vi "Cieslikiewicz_prac10.vi"() -> ()   [LabVIEW 2023]
uses:
  <vilib>/Platform/TimedLoop/XDataNode/timing_clust.ctl
  <vilib>/Platform/TimedLoop/XDataNode/nitl_modes.ctl
  <vilib>/Platform/TimedLoop/XDataNode/wakeup.ctl
  <vilib>/Platform/TimedLoop/scheduler/LVUserAPI/_suppVIs/Create_1kHz_TSource.vi
  <vilib>/platform/TimedLoop/XDataNode/XDataNode.xnode
  <vilib>/Platform/TimedLoop/XDataNode/XDNodeRunTimeDep.lvlib
panel:
  in  "Synchronizacja":bool
  out "L2 Stop":dbl
  out "Error 2":errorcluster
  out "Koniec 2":bool
  out "L2 End":dbl
  out "Numer petli 2":dbl
  out "L1 Stop":dbl
  out "czas_pocz":dbl
  out "Koniec 1":bool
  out "Error 1":errorcluster
  out "Numer petli 1":dbl
  out "L1 End":dbl
  in  "Okres (s)":dbl=0.5 min=0.5 max=20.0 step=0.5
  out "S0 End":dbl
  out "S0 Start":dbl
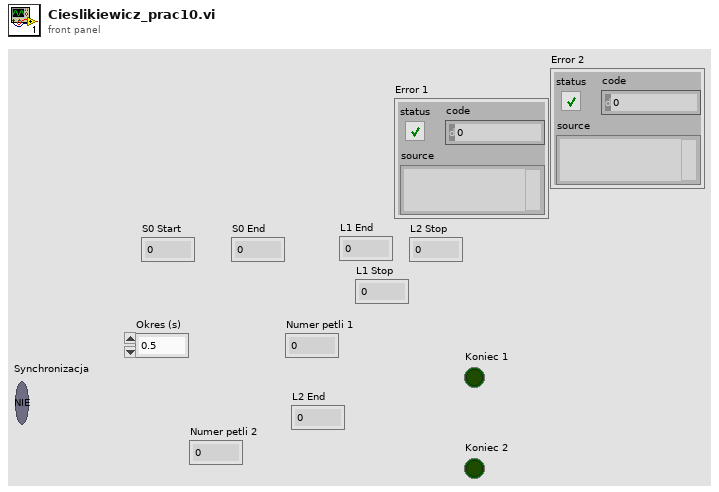
[diagram p1: front panel]
types:
  T1 = typedef "XDNodeRunTimeDep.lvlib/timing_clust.ctl" = cluster{"Expected End [f-1]":u64, "Actual End [f-1]":u64, "Finished Late? [f-1]":bool, "Expected End [i-1]":u64, "Actual End [i-1]":u64, "Finished Late? [i-1]":bool, "Expected Start [i]":u64, "Actual Start [i]":u64, "Expected Start [f]":u64, "Actual Start [f]":u64, "Source Name":string, "Structure Name":string, "Period":i64, "Deadline":i64, "Offset":i64, "Start":i64, "Priority":i32, "Timeout":i32, "Mode":T2, "Wakeup Reason":T3, "Error":errorcluster, "Source Type":string, "Secondary Source Type":string, "Global End Time":u64, "Global Start Time":u64, "Frame Duration":u64, "Iteration Duration":u64, "Assigned CPU":i32, "I/O Scan Engine Mode":u32}
  T2 = typedef "XDNodeRunTimeDep.lvlib/nitl_modes.ctl" = enum32{"No Change", "Process missed periods, maintain original phase", "Discard missed periods, maintain original phase", "Process missed periods, ignore original phase", "Discard missed periods, ignore original phase"}
  T3 = typedef "XDNodeRunTimeDep.lvlib/wakeup.ctl" = enum32{"Normal", "Aborted", "Asynchronous wakeup", "Timing source error", "Timed loop error", "Timeout"}
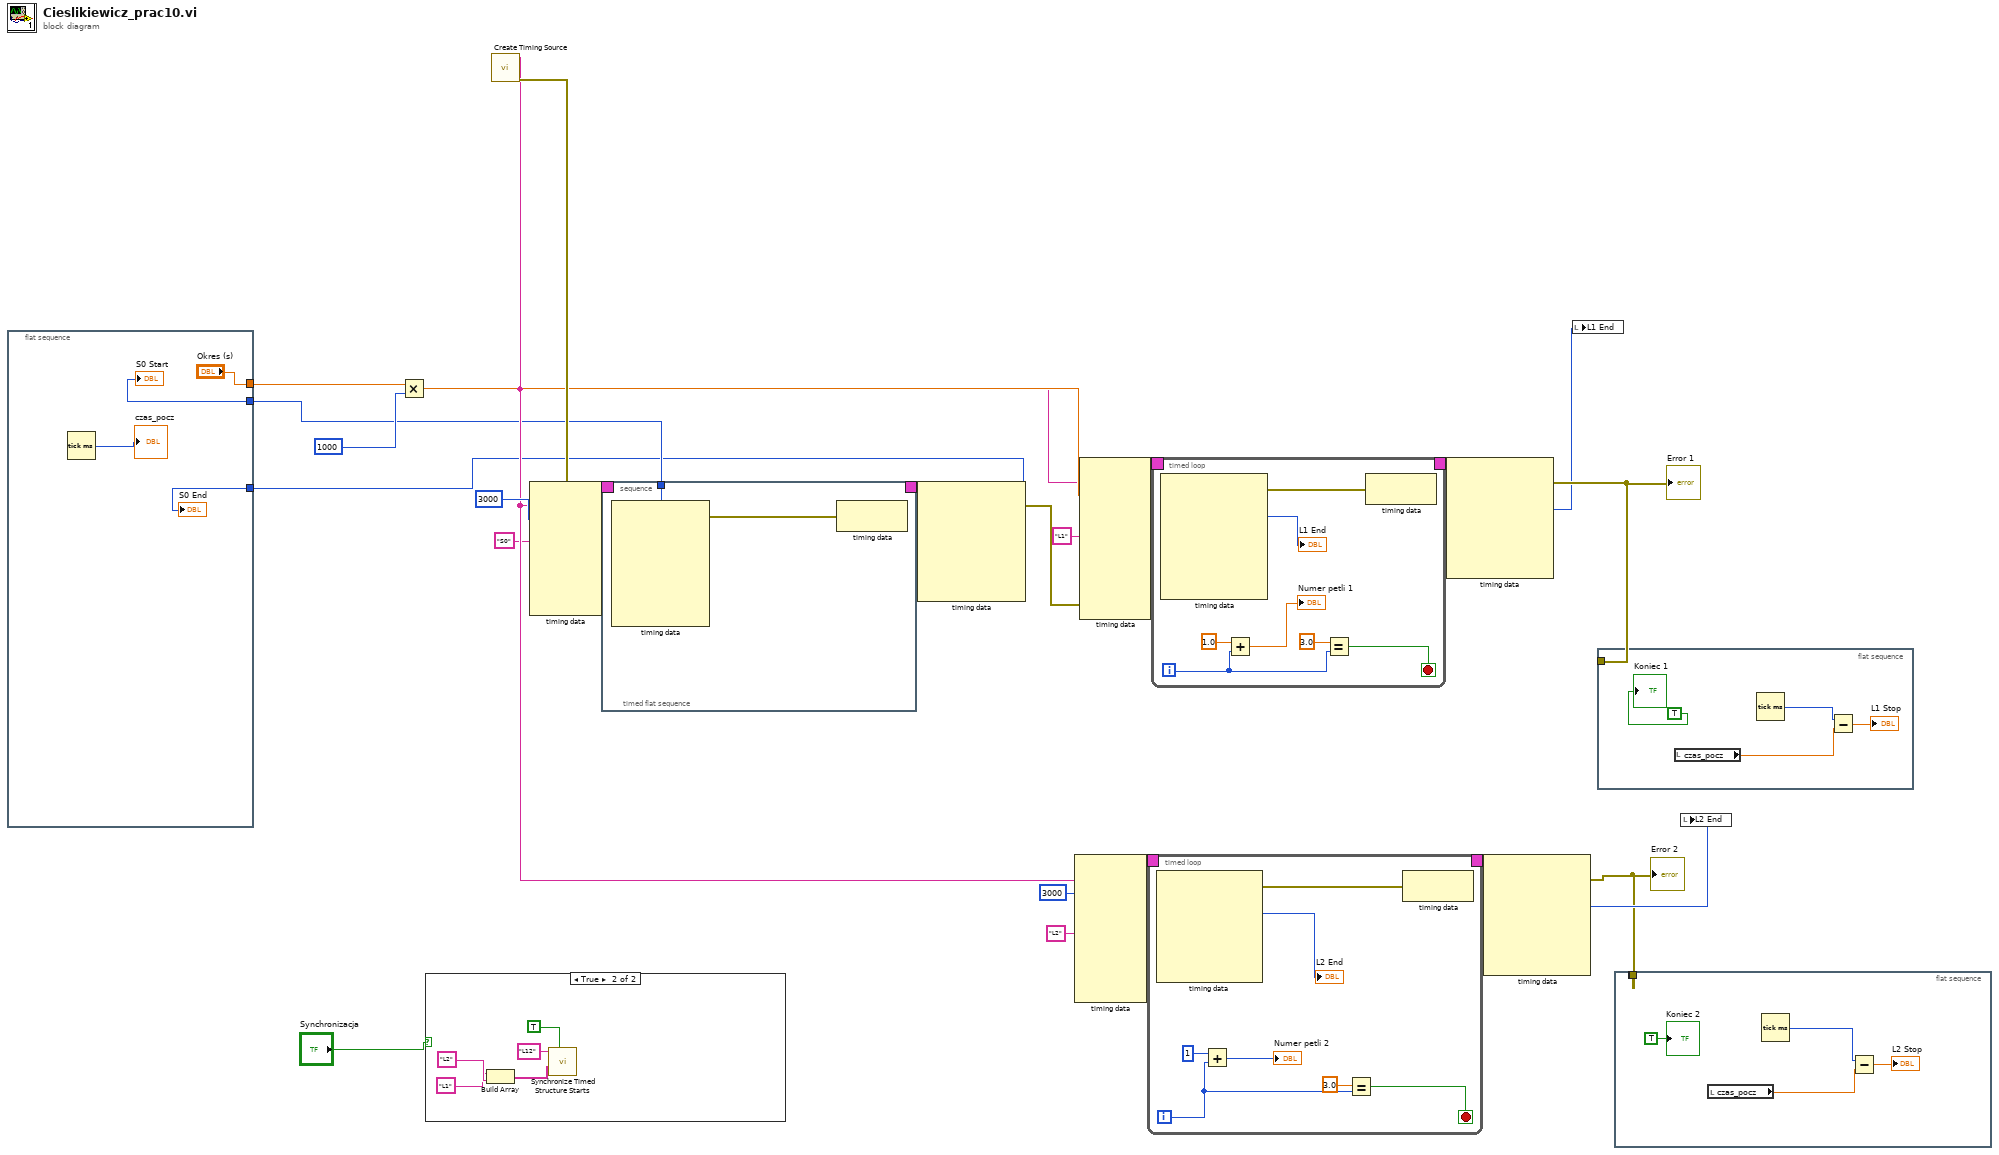
[diagram p0: block diagram]
diagram:
  n1 = flat-sequence {
    tunnel: w3 -> [w27]
    tunnel: ["Okres (s)"] -> w2
    tunnel: w1 -> [w25]
    frame #0 {
      n2 = Tick Count (ms)() -> (millisecond timer value=→"czas_pocz":u32)
      "S0 Start" <- w27
      "S0 End" <- w25
    }
  }
  n3 = Multiply(x=w2, y=1000) -> (x*y=w15:dbl)
  n4 = case shown="True" "Synchronizacja" {
    frame False {
    }
    frame True {
      n5 = Build Array("L1" ("Structure Name"), "L2" ("Structure Name")) -> (w29:string[])
      n6 = call <vilib>:"Synchronize Timed Structure Starts.vi"("replace (T)"=TRUE, "timed structure names"=w29, "synchronization group name"="L12") -> ()  [unwired: 7 in, 2 out]
    }
  }
  n7 = call-poly <vilib>:"Create Timing Source.vi"() -> ("error out"=w20:errorcluster, "name (out)"=w11:string)  [unwired: 10 in]
  n8 = node-c288(w11, i64 3000 ("Offset"), "S0" ("Structure Name"), w20) -> (w24:T1)  [unwired: 4 in]
  n9 = timed-sequence {
    timing: w24 -> [_]
    timing-out: [_] -> w23
    tunnel: [w34] -> w3
    n10 = timed-flat-sequence {
      tunnel: [w35] -> w34
      n11 = node-c288() -> (w36:errorcluster, w35:i64)  [unwired: 1 in, 6 out]
      n12 = node-c288(w36) -> ()  [unwired: 1 out]
    }
  }
  n13 = node-c288(w23) -> (w19:errorcluster, w1:i64)  [unwired: 5 out]
  n14 = node-c288(w11, i64 3000 ("Period"), "L2" ("Structure Name")) -> (w14:T1)  [unwired: 6 in]
  n15 = node-c288(w11, w15, "L1" ("Structure Name"), w19) -> (w22:T1)  [unwired: 6 in]
  n16 = timed-loop {
    timing: w14 -> [_]
    timing-out: [_] -> w13
    i -> [w46]
    stop <- w45 stop-if-true
    n17 = node-c288() -> (w44:errorcluster, →"L2 End":i64)  [unwired: 1 in, 5 out]
    n18 = Add(x=1, y=w46) -> (x+y=→"Numer petli 2":i32)
    n19 = Equal?(x=3.0, y=w46) -> (x = y?=w45:bool)
    n20 = node-c288(w44) -> ()  [unwired: 1 out]
  }
  n21 = timed-loop {
    timing: w22 -> [_]
    timing-out: [_] -> w21
    i -> [w58]
    stop <- w57 stop-if-true
    n22 = node-c288() -> (w62:errorcluster, →"L1 End":i64)  [unwired: 1 in, 6 out]
    n23 = Add(x=1.0, y=w58) -> (x+y=→"Numer petli 1":dbl)
    n24 = Equal?(x=3.0, y=w58) -> (x = y?=w57:bool)
    n25 = node-c288(w62) -> ()  [unwired: 1 out]
  }
  n26 = node-c288(w21) -> (w18:errorcluster, w10:i64)  [unwired: 5 out]
  "Error 1" <- w18
  n27 = node-c288(w13) -> (w8:errorcluster, w9:i64)  [unwired: 5 out]
  "Error 2" <- w8
  n28 = local write "L1 End"(w10) -> ()
  n29 = flat-sequence {
    tunnel: w18 -> [_]
    frame #0 {
      n30 = local read "czas_pocz"() -> (w69:dbl)
      n31 = Tick Count (ms)() -> (millisecond timer value=w70:u32)
      n32 = Subtract(x=w70, y=w69) -> (x-y=→"L1 Stop":dbl)
      "Koniec 1" <- TRUE ("Koniec")
    }
  }
  n33 = flat-sequence {
    tunnel: [w75] -> _
    tunnel: w8 -> [w75]
    frame #0 {
      n34 = local read "czas_pocz"() -> (w73:dbl)
      n35 = Tick Count (ms)() -> (millisecond timer value=w74:u32)
      n36 = Subtract(x=w74, y=w73) -> (x-y=→"L2 Stop":dbl)
      "Koniec 2" <- TRUE ("Koniec 2")
    }
  }
  n37 = local write "L2 End"(w9) -> ()
